vi "SubTemplate_4x4x4_GetClassAttributes.vi"(8 "error in (no error)":errorcluster, 11 "reference in":refnum<class "SubTemplate_4x4x4.lvclass">) -> (0 "error out":errorcluster, 1 "Attributes locked?":bool, 2 "Class attributes out":T1, 3 "reference out":refnum<class "SubTemplate_4x4x4.lvclass">)   [LabVIEW 2016, in "SubTemplate_4x4x4.lvclass"]
doc: "Returns the class attributes of this class. If reference is wired, the class attributes of the class (or sub class) will be returned else the class attributes will default to this class.\n\nIf the data is currently locked for modification, 'Attributes locked?' will return TRUE. If reference is wired, the class attributes of the class (or sub class) will be returned else the class attributes of this class."
uses:
  <resource>/Framework/Providers/Open_GDS/ClassProviders/Provider_EndevoGOOP300/Templates/SubTemplate_4x4x4/SubTemplate_4x4x4.lvclass
  <resource>/Framework/Providers/Open_GDS/ClassProviders/Provider_EndevoGOOP300/Templates/SubTemplate_4x4x4/protected/ClassAttributes.ctl
  <resource>/Framework/Providers/Open_GDS/ClassProviders/Provider_EndevoGOOP300/Templates/BaseTemplate_4x4x4/protected/ClassAttributes.ctl
  <vilib>/addons/_goop3.llb/3GOOPStates.ctl
  <resource>/Framework/Providers/Open_GDS/ClassProviders/Provider_EndevoGOOP300/Templates/BaseTemplate_4x4x4/BaseTemplate_4x4x4.lvclass
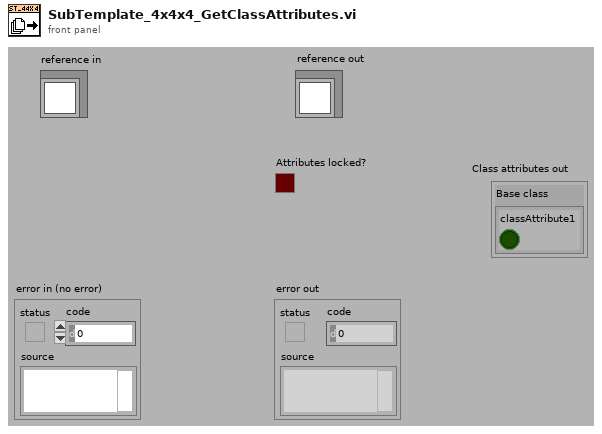
[diagram p1: front panel]
types:
  T1 = typedef "SubTemplate_4x4x4.lvclass/ClassAttributes.ctl" = cluster{"Base class":T2}
  T2 = typedef "BaseTemplate_4x4x4.lvclass/ClassAttributes.ctl" = cluster{"classAttribute1":bool}
  T3 = typedef "3GOOPStates.ctl" = enum16{"Set", "Get", "New", "Delete", "Clear", "Test and get", "Unlock data", "Information", "Look up existing", "New or look up existing", "Test and get shared", "Get shared", "Set shared", "Unlock shared", "Find dynamic method", "Register dynamic method", "Preload dynamic method", "Probe", "Cast to more generic", "Cast to more specific"}
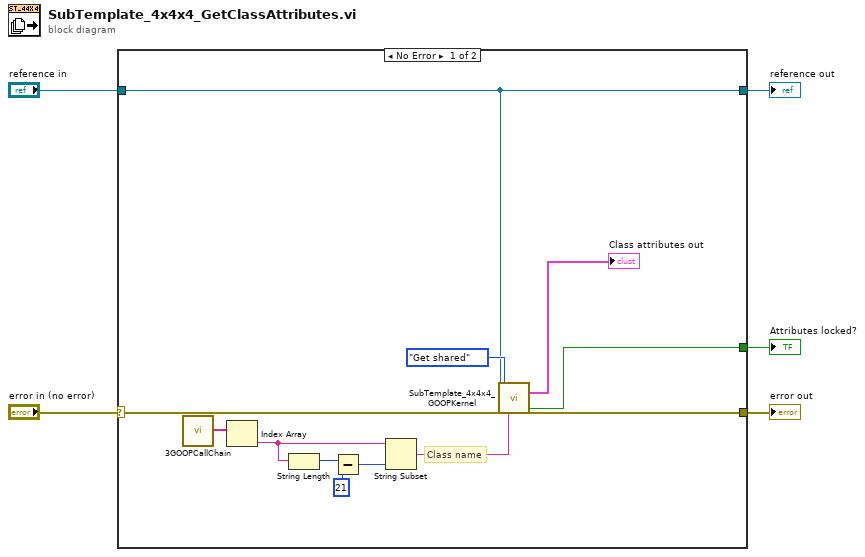
[diagram p0: block diagram]
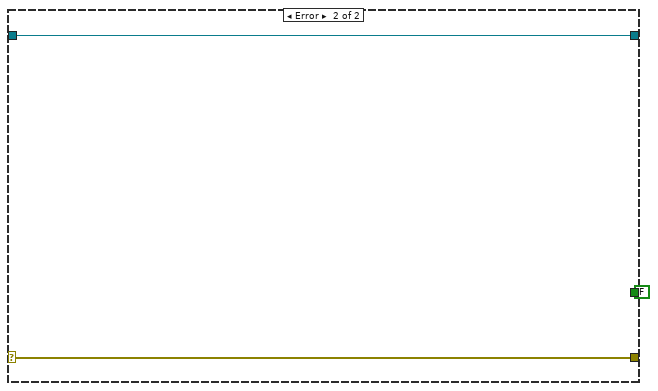
[diagram p2: hidden frame]
diagram:
  n1 = case shown="No Error" "error in (no error)" {
    selector: "error in (no error)" -> [w15 w19]
    tunnel: [w6 w20] -> w5
    tunnel: [w17 w19] -> w4
    tunnel: "reference in" -> [w6 w20]
    tunnel: [w16 FALSE ("Data locked?")] -> w1
    frame No Error {
      # "Class name"
      n2 = call <vilib>:"3GOOPCallChain.vi"() -> ("call chain"=w7:string[])
      n3 = Index Array(array=w7) -> (element=w9:string)  [unwired: 1 in]
      n4 = String Length(string=w9) -> (length=w12:i32)
      n5 = Subtract(x=w12, y=21) -> (x-y=w10:i32)
      n6 = String Subset(string=w9, length (rest)=w10) -> (substring=w8:string)  [unwired: 1 in]
      n7 = call <resource>:"SubTemplate_4x4x4_GOOPKernel.vi"("Ref in"=w6, "error in (no error)"=w15, "Action"=3GOOPStates."Get shared", "Class name"=w8) -> ("Data shared out"=→"Class attributes out":T1, "Data locked?"=w16:bool, "error out"=w17:errorcluster)  [unwired: 13 in, 8 out]
    }
    frame Error {
    }
  }
  "error out" <- w4
  "reference out" <- w5
  "Attributes locked?" <- w1
